vi "AutoHelperSequencer_ExternalStepDone_Example.vi"() -> ()   [LabVIEW 2019]
uses:
  <vilib>/Rock Robotics/WPI/ThirdParty/JAS_Junk/TrajLib/TypeDef/CHASSIS_SPEEDS.ctl
  <vilib>/Rock Robotics/WPI/ThirdParty/JAS_Junk/TrajLib/Enum/AutoHelperSequence_Step_Enum.ctl
  <vilib>/Rock Robotics/WPI/ThirdParty/JAS_Junk/TrajLib/VI/Util_GetTime_U32.vi
  <vilib>/Rock Robotics/WPI/ThirdParty/JAS_Junk/TrajLib/Timer_New.vi
  <vilib>/Rock Robotics/WPI/ThirdParty/JAS_Junk/TrajLib/VI/Util_GetTime_U64.vi
  <vilib>/Utility/semaphor.llb/Obtain Semaphore Reference.vi
  <vilib>/Rock Robotics/WPI/ThirdParty/JAS_Junk/TrajLib/Timer_Reset.vi
  <vilib>/Rock Robotics/WPI/ThirdParty/JAS_Junk/TrajLib/VI/Timer_Restart.vi
  <vilib>/Rock Robotics/WPI/ThirdParty/JAS_Junk/TrajLib/Timer_HasPeriodPassedOnce.vi
  <vilib>/Rock Robotics/WPI/ThirdParty/JAS_Junk/TrajLib/Trajectory_Library.lvlib
panel:
  out "Auto\nRunning":bool
  in  "Step 2 Done":bool
  out "Auto \nFinished":bool
  out "Elapsed Step Time":dbl
  out "Step Number State":T1
  out "Output 2":bool
  out "Output 1":bool
  out "CHASSIS\nSpeed\nDemand":T2 {"vOmega" format="%10.3f"; "vY" format="%10.3f"; "vX" format="%10.3f"}
  in  "Run Auto":bool
  out "Waveform Chart":cluster{i32, i16, i16}(graph)
  # "AUTO HELPER SEQUENCER EXAMPLE"
  # "Using external next step input"
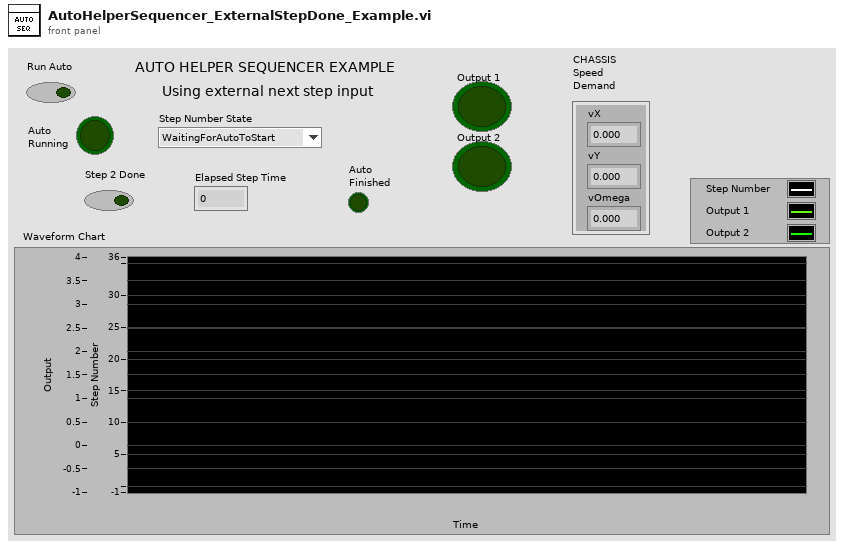
[diagram p1: front panel]
types:
  T1 = typedef "Trajectory_Library.lvlib/AutoHelperSequence_Step_Enum.ctl" = enum16{"WaitingForAutoToStart", "Step 1", "Step 2", "Step 3", "Step 4", "Step 5", "Step 6", "Step 7", "Step 8", "Step 9", "Step 10", "Step 11", "Step 12", "Step 13", "Step 14", "Step 15", "Step 16", "Step 17", "Step 18", "Step 19", "Step 20", "Step 21", "Step 22", "Step 23", "Step 24", "Step 25", "Step 26", "Step 27", "Step 28", "Step 29", "Step 30", "Step 31", "Step 32", "AutoDone"}
  T2 = typedef "Trajectory_Library.lvlib/CHASSIS_SPEEDS.ctl" = cluster{"vX":dbl, "vY":dbl, "vOmega":dbl}
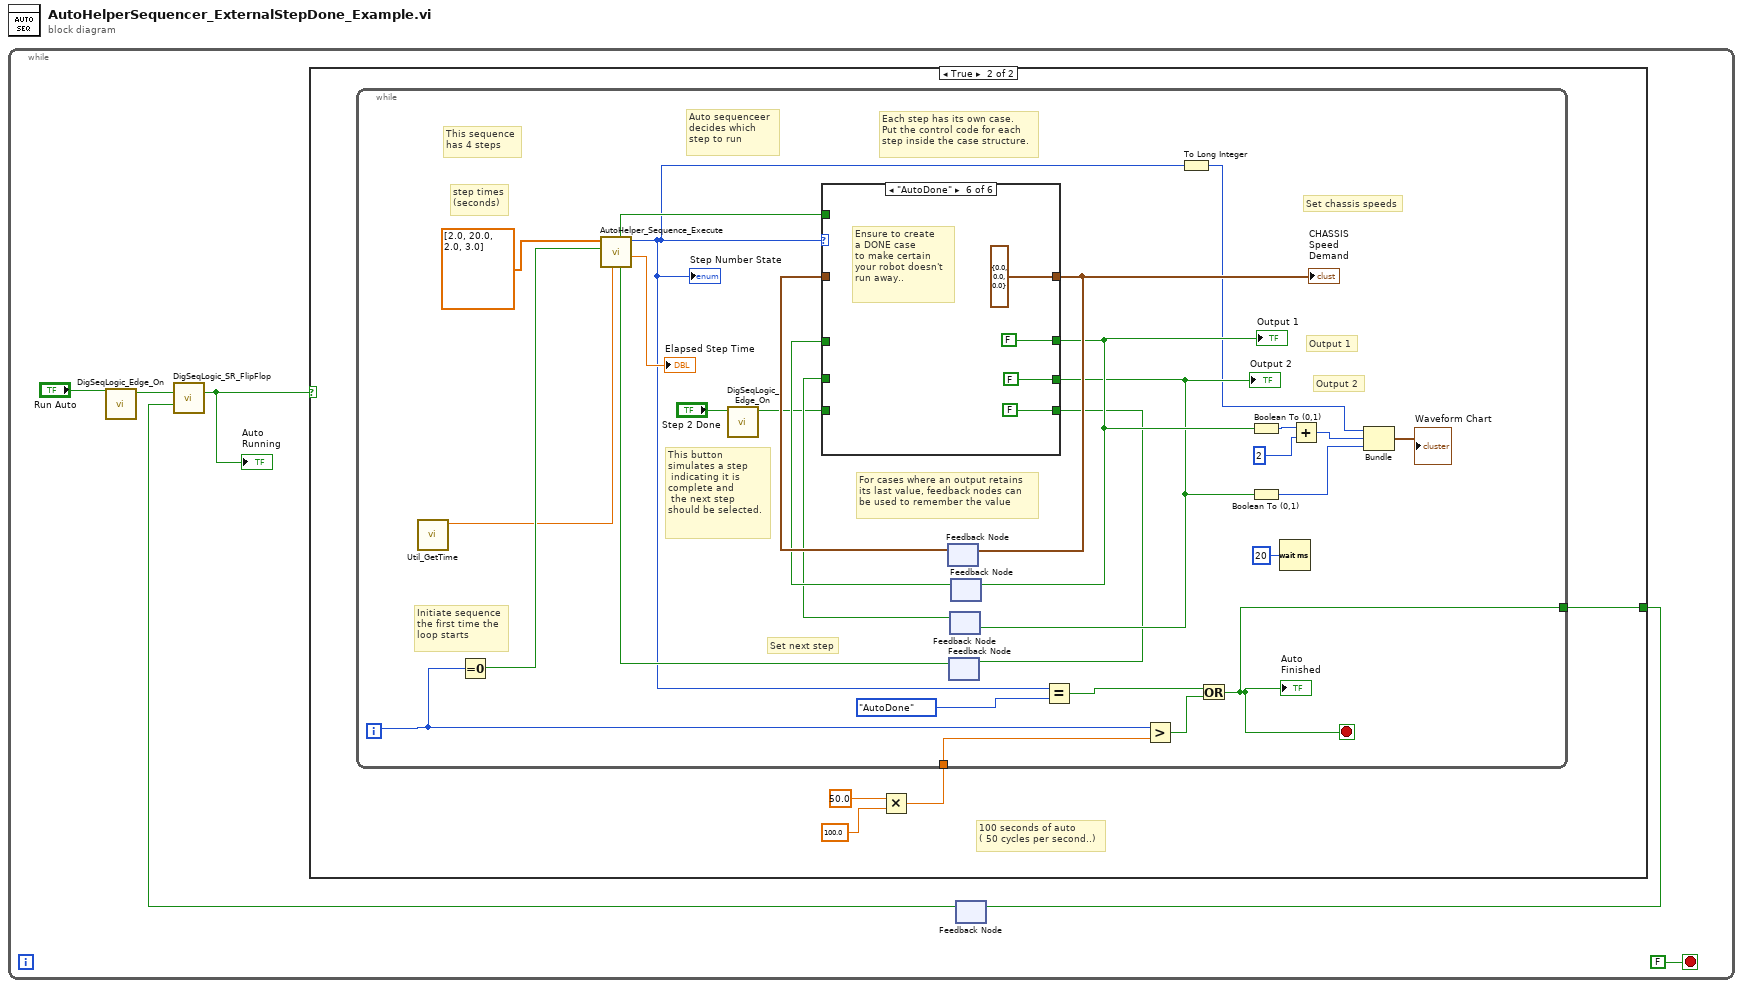
[diagram p0: block diagram]
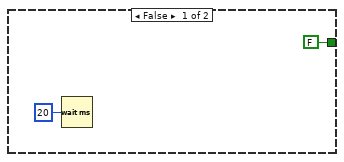
[diagram p2: hidden frame]
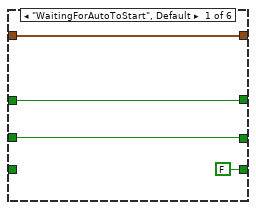
[diagram p3: hidden frame]
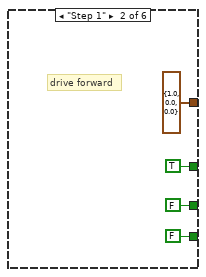
[diagram p4: hidden frame]
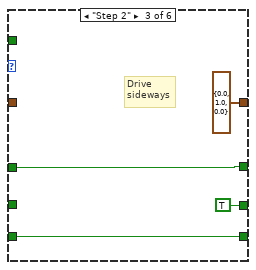
[diagram p5: hidden frame]
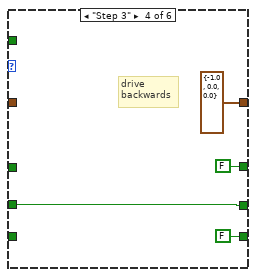
[diagram p6: hidden frame]
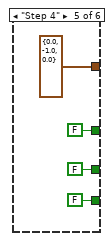
[diagram p7: hidden frame]
diagram:
  n1 = while {
    stop <- FALSE stop-if-true
    n2 = call <vilib>:"DigSeqLogic_Edge_On.vi"("Input"="Run Auto") -> ("On Edge"=w6:bool)  [unwired: 10 in]
    n3 = feedback #1() -> (w1:bool)  [unwired: 1 in]
    n4 = call <vilib>:"DigSeqLogic_SR_FlipFlop.vi"("Set"=w6, "Reset"=w1) -> ("Output"=w3:bool)  [unwired: 12 in, 1 out]
    "Auto\nRunning" <- w3
    n5 = case shown="True" w3 {
      tunnel: [FALSE w9] -> w2
      frame False {
        n6 = Wait (ms)(milliseconds to wait=u32 20) -> ()  [unwired: 1 out]
      }
      frame True {
        # "100 seconds of auto\n( 50 cycles per second..)"
        n7 = Multiply(x=50.0, y=100.0) -> (x*y=w10:dbl)
        n8 = while {
          tunnel: w10 -> [w23]
          tunnel: [w13] -> w9
          i -> [w24]
          stop <- w13 stop-if-true
          # "This button \nsimulates a step\n indicating it is\ncomplete and\n the next step \nshould be selected."
          # "Set next step"
          # "step times\n(seconds)"
          # "This sequence\nhas 4 steps"
          # "Set chassis speeds"
          # "For cases where an output retains\nits last value, feedback nodes can \nbe used to remember the value"
          # "Output 2"
          # "Output 1"
          # "Each step has its own case.\nPut the control code for each\nstep inside the case structure."
          # "Auto sequenceer\ndecides which\nstep to run"
          # "Initiate sequence\nthe first time the \nloop starts"
          n9 = call <vilib>:"Util_GetTime.vi"() -> ("FPGA_Time_Seconds"=w33:dbl)  [unwired: 9 in, 2 out]
          n10 = Equal To 0?(x=w24) -> (x = 0?=w34:bool)
          n11 = call <vilib>:"DigSeqLogic_Edge_On.vi"("Input"="Step 2 Done") -> ("On Edge"=w21:bool)  [unwired: 10 in]
          n12 = feedback #2() -> (w31:T2)  [unwired: 1 in]
          n13 = feedback #3() -> (w19:bool)  [unwired: 1 in]
          n14 = call <vilib>:"AutoHelper_Sequence_Execute.vi"("Set Next Step"=w19, "Pass_Through_Time"=w33, "Initiate"=w34, "Step Times Sec"=dbl[] [2.0, 20.0, 2.0, 3.0]) -> ("Elapsed Step Time"=→"Elapsed Step Time":dbl, "Step Number State"=w15:T1, "New Step"=w26:bool)  [unwired: 3 in, 2 out]
          "Step Number State" <- w15
          n15 = feedback #4() -> (w29:bool)  [unwired: 1 in]
          n16 = feedback #5() -> (w30:bool)  [unwired: 1 in]
          n17 = case shown="\"AutoDone\"" w15 {
            tunnel: [w44 TRUE w53 FALSE FALSE FALSE] -> w28
            tunnel: [w45 T2 {"vX"=1.0, "vY"=0.0, "vOmega"=0.0} T2 {"vX"=0.0, "vY"=1.0, "vOmega"=0.0} T2 {"vX"=-1.0, "vY"=0.0, "vOmega"=0.0} T2 {"vX"=0.0, "vY"=-1.0, "vOmega"=0.0} T2 {"vX"=0.0, "vY"=0.0, "vOmega"=0.0}] -> w32
            tunnel: [w43 FALSE TRUE w56 FALSE FALSE] -> w27
            tunnel: w31 -> [w45 _ _ _ _ _]
            tunnel: w30 -> [w44 _ w53 _ _ _]
            tunnel: w29 -> [w43 _ _ w56 _ _]
            tunnel: w26 -> [_ _ _ _ _ _]
            tunnel: [FALSE ("On Edge") FALSE ("On Edge") w50 FALSE ("On Edge") FALSE ("On Edge") FALSE ("On Edge")] -> w20
            tunnel: w21 -> [_ _ w50 _ _ _]
            frame "WaitingForAutoToStart", Default {
            }
            frame "Step 1" {
              # "drive forward"
            }
            frame "Step 2" {
              # "Drive \nsideways"
            }
            frame "Step 3" {
              # "drive\nbackwards"
            }
            frame "Step 4" {
            }
            frame "AutoDone" {
              # "Ensure to create\na DONE case\nto make certain\nyour robot doesn't\nrun away.."
            }
          }
          "CHASSIS\nSpeed\nDemand" <- w32
          "Output 1" <- w28
          "Output 2" <- w27
          n18 = feedback-in #2(w32) -> ()
          n19 = feedback-in #3(w20) -> ()
          n20 = feedback-in #4(w27) -> ()
          n21 = feedback-in #5(w28) -> ()
          n22 = Equal?(x=w15, y=AutoHelperSequence_Step_Enum."AutoDone" ("Step Number State")) -> (x = y?=w17:bool)
          n23 = Greater?(x=w24, y=w23) -> (0:w16:bool)
          n24 = To Long Integer(number=w15) -> (32bit integer=w14:i32)
          n25 = Or(x=w17, y=w16) -> (x .or. y?=w13:bool)
          "Auto \nFinished" <- w13
          n26 = Boolean To (0,1)(Boolean=w28) -> (0, 1=w38:i16)
          n27 = Boolean To (0,1)(Boolean=w27) -> (0, 1=w36:i16)
          n28 = Wait (ms)(milliseconds to wait=u32 20) -> ()  [unwired: 1 out]
          n29 = Add(x=w38, y=i16 2) -> (x+y=w37:i16)
          n30 = Bundle(w14, w37, w36) -> (→"Waveform Chart":cluster{i32, i16, i16})  [unwired: 1 in]
        }
      }
    }
    n31 = feedback-in #1(w2) -> ()
  }
